vi "Configure Trigger Model Measure Block.vi"(8 "error in (no error)":errorcluster, 9 "Buffer Name (defbuffer1)":string="defbuffer1", 10 "Block Number (1)":i32=1 min=1 format="%#.6g", 11 "VISA resource name":refnum<visa-resource-name>) -> (0 "error out":errorcluster, 3 "VISA resource name out":refnum<visa-resource-name>)   [LabVIEW 2017, in "Keithley 2450.lvlib"]
doc: "This VI defines a trigger block that makes a measurement.The trigger model waits for the measurement to complete.The instrument places the measurement into the specified reading buffer. If no buffer is specified, the reading is placed into the default buffer (defbuffer1)."
uses:
  Keithley 2450.lvlib
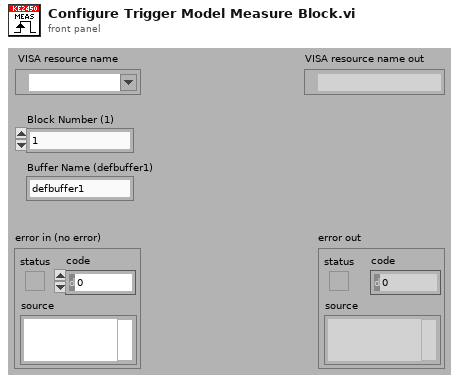
[diagram p1: front panel]
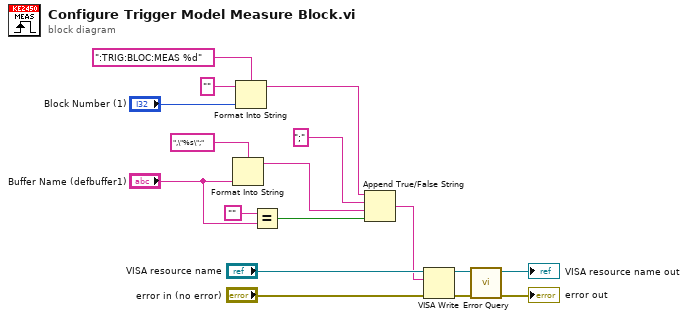
[diagram p0: block diagram]
diagram:
  n1 = Format Into String(format string=",\"%s\";", "Buffer Name (defbuffer1)") -> (resulting string=w4:string)  [unwired: 2 in, 1 out]
  n2 = Format Into String(format string=":TRIG:BLOC:MEAS %d", initial string="", "Block Number (1)") -> (resulting string=w2:string)  [unwired: 1 in, 1 out]
  n3 = Equal?(x="" ("y"), y="Buffer Name (defbuffer1)") -> (x = y?=w3:bool)
  n4 = Append True/False String(1:w3, 2:w4, 3:";" ("true string"), 4:w2) -> (0:w5:string)
  n5 = VISA Write(VISA resource name="VISA resource name", write buffer=w5, error in (no error)="error in (no error)") -> (VISA resource name out=w13:refnum<visa-resource-name>, error out=w12:errorcluster)  [unwired: 1 out]
  n6 = call "Error Query.vi"("error in (no error)"=w12, "VISA resource name"=w13) -> ("error out"=→"error out":errorcluster, "VISA resource name out"=→"VISA resource name out":refnum<visa-resource-name>)  [unwired: 8 out]
